vi "ECOG-Update Spectrogram.vi"(0 "new data":dbl[](array[numeric]), 11 "spectrogram in":T1) -> (4 "new data thru":dbl[](array[numeric]), 15 "spectrogram out":T1)   [LabVIEW 2020]
uses:
  Typedefs/ECOG-Spectrogram.ctl
  5e1dc45d-3397-4ae4-9168-812a6a074c8d.vi
  <vilib>/Analysis/baseanly.llb/Mean.vi
  <vilib>/Analysis/baseanly.llb/Mean (DBL).vi
  epl-vi-lib/Utility VIs/Array Manipulation VIs/Array-Dimensions (2D).vi
  epl-vi-lib/Utility VIs/Math VIs/FFTtoR,Theta (1D).VI
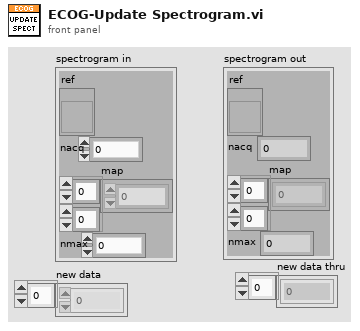
[diagram p1: front panel]
types:
  T1 = typedef "ECOG-Spectrogram.ctl" = cluster{"ref":refnum<vi>, "nacq":i32, "map":dbl[][], "nmax":i32}
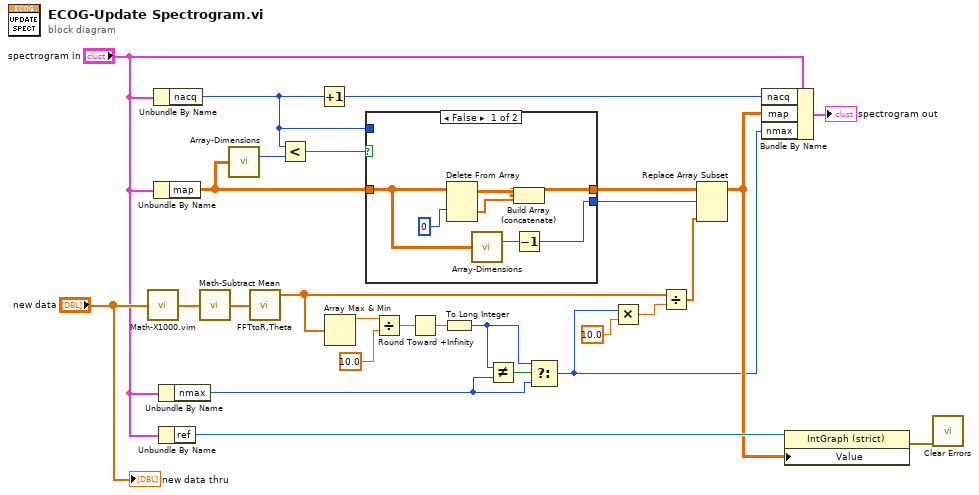
[diagram p0: block diagram]
diagram:
  n1 = call "Math-X1000.vim"("X"="new data") -> ("1000X"=w9:dbl[])
  n2 = Unbundle By Name("spectrogram in") -> ("nacq"=w24:i32)
  n3 = Unbundle By Name("spectrogram in") -> ("map"=w19:dbl[][])
  n4 = Unbundle By Name("spectrogram in") -> ("nmax"=w2:i32)
  n5 = Unbundle By Name("spectrogram in") -> ("ref"=w22:refnum<vi>)
  n6 = call "Math-Subtract Mean.vi"("Y"=w9) -> ("Y - mean(Y)"=w17:dbl[])  [unwired: 4 in]
  n7 = call-poly "Array-Dimensions.vi"("2D Array"=w19) -> ("# rows"=w16:i32)  [unwired: 13 in, 1 out]
  n8 = call-poly "FFTtoR,Theta.VI"("X"=w17) -> ("+Freq. Mag of FFT"=w8:dbl[])  [unwired: 1 in, 1 out]
  n9 = Less?(x=w24, y=w16) -> (x < y?=w27:bool)
  n10 = Increment(x=w24) -> (x+1=w26:i32)
  n11 = Array Max & Min(array=w8) -> (max value=w10:dbl)  [unwired: 3 out]
  n12 = case shown="False" w27 {
    tunnel: w19 -> [w28 w36]
    tunnel: [w29 w36] -> w25
    tunnel: w24 -> [_ w35]
    tunnel: [w33 w35] -> w23
    frame False {
      n13 = Delete From Array(array=w28, index (row)=0) -> (deleted portion=w30:dbl[], array with subset deleted=w32:dbl[][])  [unwired: 2 in]
      n14 = call-poly "Array-Dimensions.vi"("2D Array"=w28) -> ("# rows"=w31:i32)  [unwired: 13 in, 1 out]
      n15 = Build Array (concatenate)(w32, w30) -> (w29:dbl[][])
      n16 = Decrement(x=w31) -> (x-1=w33:i32)
    }
    frame True {
    }
  }
  n17 = Divide(x=w10, y=10.0) -> (x/y=w12:dbl)
  n18 = Round Toward +Infinity(x=w12) -> (ceil(x): smallest int >= x=w13:dbl)
  n19 = To Long Integer(number=w13) -> (32bit integer=w3:i32)
  n20 = Not Equal?(x=w3, y=w2) -> (x != y?=w4:bool)
  n21 = Select(t=w3, s=w4, f=w2) -> (s? t:f=w1:i32)
  n22 = Multiply(x=w1, y=10.0) -> (x*y=w6:dbl)
  n23 = Divide(x=w8, y=w6) -> (x/y=w14:dbl[])
  n24 = Replace Array Subset(array=w25, new element=w14, index (row)=w23) -> (w15:dbl[][])  [unwired: 1 in]
  n25 = Bundle By Name(cluster="spectrogram in", "nacq"=w26, "map"=w15, "nmax"=w1) -> (→"spectrogram out":T1)
  n26 = property class="IntGraph (strict)"(reference=w22, "Value"=w15) -> (error out=w20:errorcluster)  [unwired: 1 in, 1 out]
  n27 = call <vilib>:"Clear Errors.vi"("error in (no error)"=w20) -> ()  [unwired: 5 in, 2 out]
  "new data thru" <- "new data"
